vi "sample10(DXL).vi"() -> ()   [LabVIEW 2011]
panel:
  in  "Baudrate":u32=57600 min=9600 max=12000000
  in  "COM":refnum<visa-resource-name> caption="COMポート"
  out "ids":u8[](array[numeric])
  in  "angle":dbl(knob) scale=-180.0..180.0
  in  "停止":bool
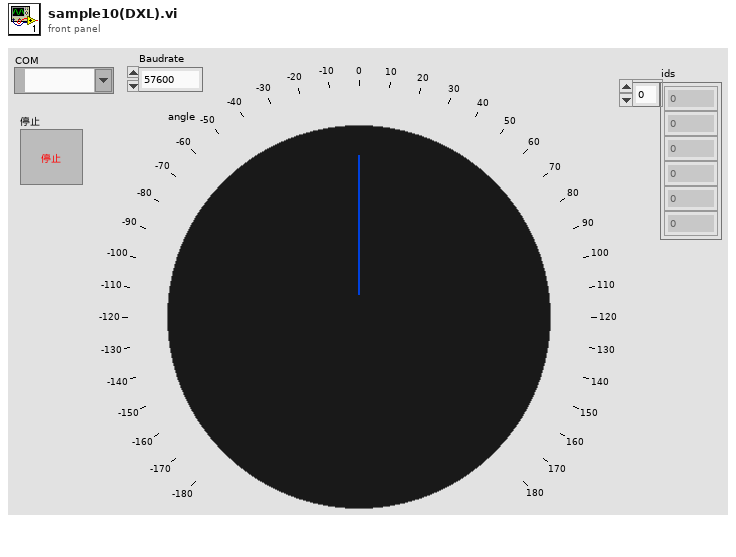
[diagram p1: front panel]
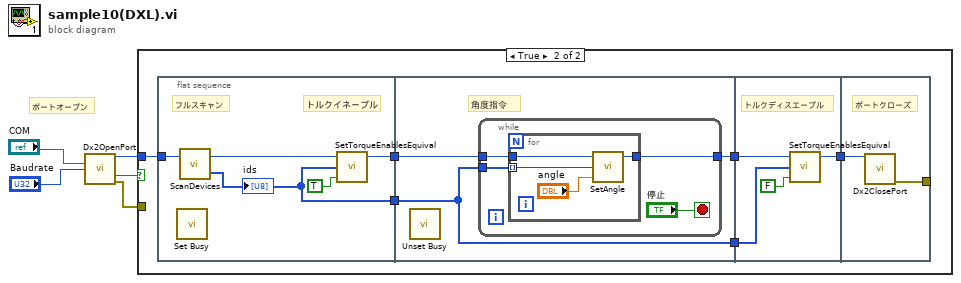
[diagram p0: block diagram]
diagram:
  # "ポートオープン"
  n1 = call "Dx2OpenPort.vi"("port"="COM", "baudrate"="Baudrate") -> ("dvid"=w4:u32, "成功"=w5:bool, "エラー出力"=w3:errorcluster)  [unwired: 11 in]
  n2 = case shown="TRUE" w5 {
    tunnel: w4 -> [_ w11]
    tunnel: w3 -> [_ _]
    frame False {
    }
    frame True {
      n3 = flat-sequence {
        tunnel: [w13] -> w10
        tunnel: w11 -> [w16]
        tunnel: [w12] -> w9
        tunnel: w10 -> [w19]
        tunnel: [w18] -> w8
        tunnel: w9 -> [w17]
        tunnel: [w17] -> w6
        tunnel: w8 -> [w29]
        tunnel: [w30] -> w7
        tunnel: w6 -> [w28]
        tunnel: [w32] -> _
        tunnel: w7 -> [w33]
        frame #0 {
          # "トルクイネーブル"
          # "フルスキャン"
          n4 = call <vilib>:"Set Busy.vi"() -> ()  [unwired: 10 in, 2 out]
          n5 = call "ScanDevices.vi"("dvid in"=w16) -> ("ids"=w12:u8[], "dvid out"=w15:u32)  [unwired: 1 in]
          "ids" <- w12
          n6 = call "SetTorqueEnablesEquival.vi"("torqueenable"=TRUE, "ids"=w12, "dvid in"=w15) -> ("dvid out"=w13:u32)  [unwired: 1 in, 1 out]
        }
        frame #1 {
          # "角度指令"
          n7 = call <vilib>:"Unset Busy.vi"() -> ()  [unwired: 11 in, 1 out]
          n8 = while {
            tunnel: w19 -> [w23]
            tunnel: [w21] -> w18
            tunnel: w17 -> [w20]
            stop <- "停止" stop-if-true
            n9 = for {
              tunnel: w23 -> [w27]
              tunnel: [w25] -> w21
              tunnel: w20 -> [w24] mode=indexing
              n10 = call "SetAngle.vi"("angle"="angle", "Target ID"=w24, "dvid in"=w27) -> ("dvid out"=w25:u32)  [unwired: 1 in, 1 out]
            }
          }
        }
        frame #2 {
          # "トルクディスエーブル"
          n11 = call "SetTorqueEnablesEquival.vi"("torqueenable"=FALSE, "ids"=w28, "dvid in"=w29) -> ("dvid out"=w30:u32)  [unwired: 1 in, 1 out]
        }
        frame #3 {
          # "ポートクローズ"
          n12 = call "Dx2ClosePort.vi"("dvid"=w33) -> ("エラー出力"=w32:errorcluster)  [unwired: 13 in, 1 out]
        }
      }
    }
  }
